vi "Execute default event by ID.vi"(6 "Event Name":string, 8 "Module ID":i32, 9 "Module type":T1, 10 "Module Lib":refnum<vi>, 11 "References Map":map{string, refnum<vi>}(c390)) -> (0 "error out":errorcluster)   [LabVIEW 2020, in "Panter Dashboard.lvlib"]
uses:
  Panter Dashboard.lvlib
  Module type--enum.ctl
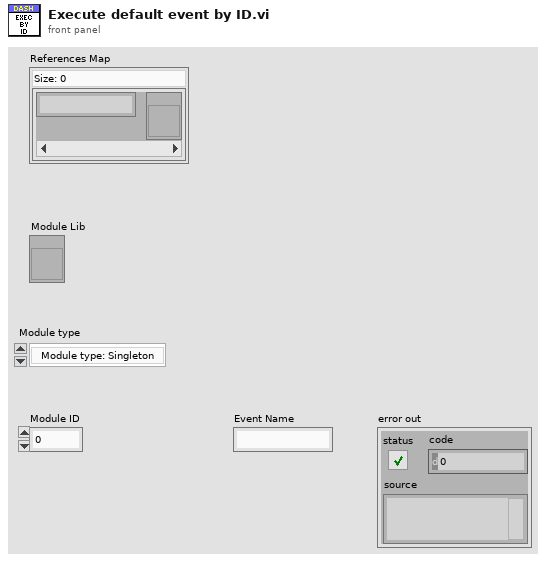
[diagram p1: front panel]
types:
  T1 = typedef "Panter Dashboard.lvlib/Module type--enum.ctl" = enum16{"Module type: Singleton", "Module type: Cloneable"}
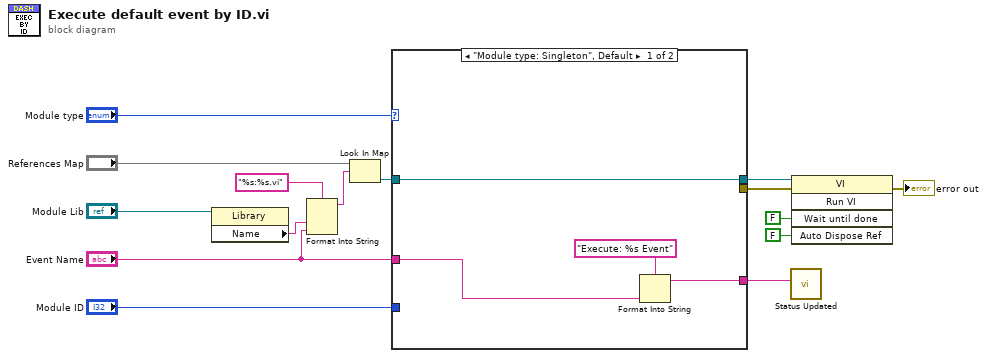
[diagram p0: block diagram]
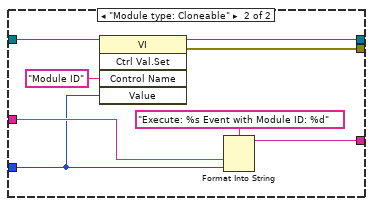
[diagram p2: hidden frame]
diagram:
  n1 = property class="Library"(reference="Module Lib") -> ("Name"=w4:string)  [unwired: 1 in, 2 out]
  n2 = Format Into String(format string="%s:%s.vi", w4, "Event Name") -> (resulting string=w10:string)  [unwired: 2 in, 1 out]
  n3 = Look In Map(map="References Map", key=w10) -> (value=w8:refnum<vi>)  [unwired: 1 in, 1 out]
  n4 = case shown="\"Module type: Singleton\", Default" "Module type" {
    tunnel: [_ w27] -> w14
    tunnel: w8 -> [w19 w26]
    tunnel: "Module ID" -> [_ w22]
    tunnel: [w19 w24] -> w6
    tunnel: "Event Name" -> [w18 w23]
    tunnel: [w17 w21] -> w1
    frame "Module type: Singleton", Default {
      n5 = Format Into String(format string="Execute: %s Event", w18) -> (resulting string=w17:string)  [unwired: 2 in, 1 out]
    }
    frame "Module type: Cloneable" {
      n6 = invoke class="VI" method="Ctrl Val.Set"(reference=w26, "Control Name"="Module ID", "Value"=w22) -> (reference out=w24:refnum<vi>, error out=w27:errorcluster)  [unwired: 2 in, 3 out]
      n7 = Format Into String(format string="Execute: %s Event with Module ID: %d", w23, w22) -> (resulting string=w21:string)  [unwired: 2 in, 1 out]
    }
  }
  n8 = call "Status Updated.vi"("Status"=w1) -> ()  [unwired: 10 in, 1 out]
  n9 = invoke class="VI" method="Run VI"(reference=w6, error in=w14, "Wait until done"=FALSE ("Wait Until Done"), "Auto Dispose Ref"=FALSE ("Auto Dispose Reference")) -> (error out=→"error out":errorcluster)  [unwired: 1 in, 4 out]
